vi "JSONtext and SQlite (requires SQLite LabVIEW).vi"() -> ()   [LabVIEW 2017]
uses:
  <vilib>/drjdpowell/SQLite Library/SQL Statement/SQL Statement.lvclass/SQL Statement.ctl
  <vilib>/drjdpowell/SQLite Library/SQL Connection/Open (path).vi
  <vilib>/drjdpowell/SQLite Library/SQL Statement/Bind UTF-8 Text.vi
  a4ef3bbe-680b-444f-9f5b-3aba932734da.vi
  <vilib>/drjdpowell/SQLite Library/SQL Statement/Bind Integer.vi
  <vilib>/drjdpowell/SQLite Library/SQL Connection/Open (string).vi
  <vilib>/AdvancedString/Path To Command Line String.vi
  <vilib>/drjdpowell/SQLite Library/SQL Connection/Execute SQL (No results).vi
  <vilib>/drjdpowell/SQLite Library/SQL Statement/Error Message.vi
  <vilib>/drjdpowell/SQLite Library/SQL Connection/Execute SQL (Single DBL).vi
  <vilib>/drjdpowell/SQLite Library/SQL Statement/Column UTF-8 Text.vi
  JSON text to Variant.vi
  <vilib>/drjdpowell/SQLite Library/SQL Connection/Connection.lvclass
  JSONtext.lvlib
  <vilib>/drjdpowell/SQLite Library/SQLite.lvlib
  <vilib>/drjdpowell/SQLite Library/SQL Statement/SQL Statement.lvclass
  <vilib>/drjdpowell/SQLite Library/Transaction Helpers/Transaction.lvlib
panel:
  out "Average Age":dbl format="%#.6g"
  out "Returned":cluster{string, dbl, string}[](array[cluster]) caption="Returned people of that age" {"?" format="%#_f"}
  in  "Age":i64=32
  # "This example requires both JSONtext and \"SQLite LabVIEW\" packages"
  # "http://sine.ni.com/nips/cds/view/p/lang/en/nid/212894"
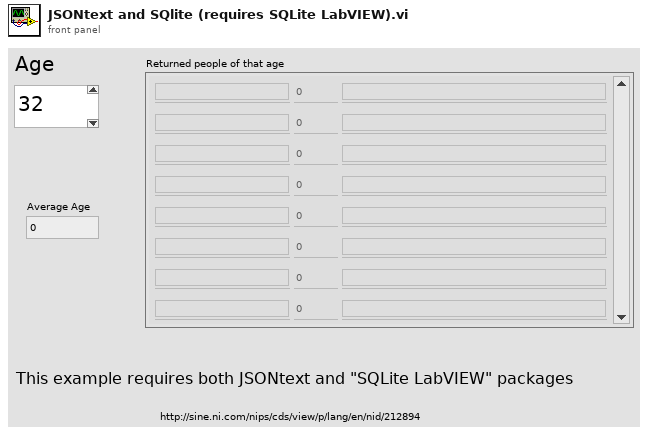
[diagram p1: front panel]
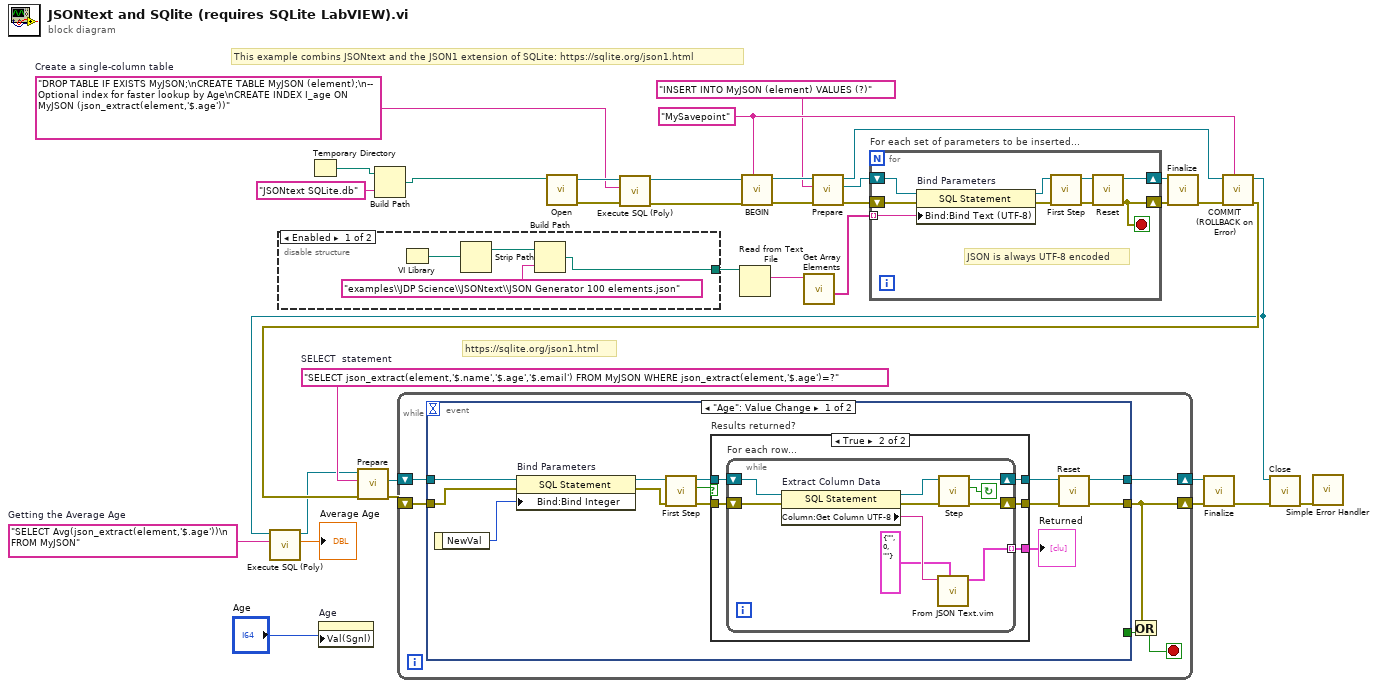
[diagram p0: block diagram]
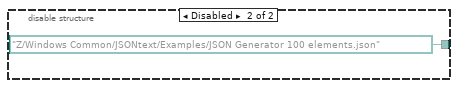
[diagram p2: hidden frame]
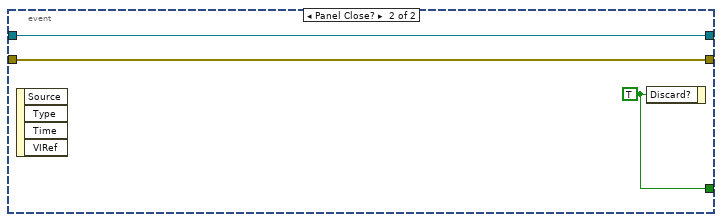
[diagram p4: hidden frame]
diagram:
  w6 = "SELECT Avg(json_extract(element,'$.age'))\n FROM MyJSON"  # Getting the Average Age
  w14 = "SELECT json_extract(element,'$.name','$.age','$.email') FROM MyJSON WHERE json_extract(element,'$.age')=?"  # SELECT  statement
  w29 = "MySavepoint" ("Savepoint name")
  w32 = "DROP TABLE IF EXISTS MyJSON;\nCREATE TABLE MyJSON (element);\n-- Optional index for faster lookup by Age\nCREATE INDEX I_age ON MyJSON (json_extract(element,'$.age'))"  # Create a single-column table
  # "This example combins JSONtext and the JSON1 extension of SQLite: https://sqlite.org/json1.html"
  # "https://sqlite.org/json1.html"
  n1 = disable-structure shown="Enabled" {
    disable-tunnel: [w35 path "Z:/Windows Common/JSONtext/Examples/JSON Generator 100 elements.json" ("appended path")] -> w1
    frame Enabled {
      n2 = VI Library() -> (path=w37:path)
      n3 = Strip Path(path=w37) -> (stripped path=w38:path)  [unwired: 1 out]
      n4 = Build Path(base path=w38, name or relative path="examples\\JDP Science\\JSONtext\\JSON Generator 100 elements.json") -> (appended path=w35:path)
    }
    frame Disabled {
    }
  }
  n5 = Temporary Directory() -> (w4:path)
  n6 = property on="Age" class="DigNum (strict)"("Val(Sgnl)"="Age") -> ()  [unwired: 2 in, 2 out]
  n7 = Build Path(base path=w4, name or relative path="JSONtext SQLite.db") -> (appended path=w2:path)
  n8 = call-poly <vilib>:"Open.vi"("db file"=w2) -> ("error out"=w19:errorcluster, "SQLite Connection"=w33:refnum<class "Connection.lvclass">)  [unwired: 9 in]
  n9 = call-poly <vilib>:"Execute SQL (Poly).vi"("error in (no error)"=w19, "SQL"=w32, "SQLite Connection in"=w33) -> ("error out"=w18:errorcluster, "SQLite Connection"=w20:refnum<class "Connection.lvclass">)  [unwired: 7 in]
  n10 = Read from Text File(file (use dialog)=w1) -> (text=w34:string)  [unwired: 3 in, 3 out]
  n11 = call <vilib>:"BEGIN.vi"("Savepoint name"=w29, "error in (no error)"=w18, "SQLite Connection in"=w20) -> ("error out"=w28:errorcluster, "SQLite Connection"=w27:refnum<class "Connection.lvclass">)  [unwired: 7 in]
  n12 = call "Get Array Elements.vi"("JSON"=w34) -> ("<JSON>"=w21:string[])  [unwired: 8 in, 2 out]
  n13 = call <vilib>:"Prepare.vi"("error in (no error)"=w28, "SQL"="INSERT INTO MyJSON (element) VALUES (?)" ("INSERT statement"), "SQLite Connection in"=w27) -> ("error out"=w23:errorcluster, "SQL Statement"=w22:refnum<class "SQL Statement.lvclass">, "SQLite Connection"=w30:refnum<class "Connection.lvclass">)  [unwired: 4 in, 2 out]
  n14 = for "For each set of parameters to be inserted..." {
    shift-right: [w42] -> w25
    shift-left: w22 -> [w48]
    shift-right: [w41] -> w26
    shift-left: w23 -> [w45]
    tunnel: w21 -> [w40] mode=indexing
    stop <- w41 stop-if-true
    # "JSON is always UTF-8 encoded"
    n15 = property on="Bind Parameters" class="SQL Statement"(reference=w48, error in=w45, "Bind:Bind Text (UTF-8)"=w40) -> (reference out=w47:refnum<class "SQL Statement.lvclass">, error out=w46:errorcluster)
    n16 = call <vilib>:"First Step.vi"("error in (no error)"=w46, "SQL Statement in"=w47) -> ("error out"=w44:errorcluster, "SQL Statement"=w43:refnum<class "SQL Statement.lvclass">)  [unwired: 7 in, 1 out]
    n17 = call <vilib>:"Reset.vi"("error in (no error)"=w44, "SQL Statement in"=w43) -> ("error out"=w41:errorcluster, "SQL Statement"=w42:refnum<class "SQL Statement.lvclass">)  [unwired: 8 in]
  }
  n18 = call <vilib>:"Finalize.vi"("error in (no error)"=w26, "SQL Statement in"=w25) -> ("error out"=w31:errorcluster)  [unwired: 9 in]
  n19 = call <vilib>:"COMMIT (ROLLBACK on Error).vi"("Savepoint name"=w29, "error in (no error)"=w31, "SQLite Connection in"=w30) -> ("error out"=w10:errorcluster, "SQLite Connection"=w7:refnum<class "Connection.lvclass">)  [unwired: 7 in]
  n20 = call-poly <vilib>:"Execute SQL (Poly).vi"("SQL"=w6, "SQLite Connection in"=w7) -> ("Result"=→"Average Age":dbl, "SQLite Connection"=w8:refnum<class "Connection.lvclass">)  [unwired: 7 in, 1 out]
  n21 = call <vilib>:"Prepare.vi"("error in (no error)"=w10, "SQL"=w14, "SQLite Connection in"=w8) -> ("error out"=w13:errorcluster, "SQL Statement"=w12:refnum<class "SQL Statement.lvclass">)  [unwired: 4 in, 3 out]
  n22 = while {
    shift-right: [w49] -> w16
    shift-left: w13 -> [w53]
    shift-right: [w54] -> w15
    shift-left: w12 -> [w52]
    stop <- w50 stop-if-true
    n23 = event shown="[0] \"Age\": Value Change" {
      selector: _ -> [_ _]
      dyn-events: _ -> [_ _]
      timeout: _ -> [_ _]
      tunnel: [w57 w85] -> w49
      tunnel: [w56 w86] -> w54
      tunnel: w53 -> [w67 w85]
      tunnel: w52 -> [w64 w86]
      tunnel: [_ w87] -> w51
      event "Age": Value Change {
        n24 = event-data() -> ("NewVal"=w60:i64)  [unwired: 1 in]
        n25 = property on="Bind Parameters" class="SQL Statement"(reference=w64, error in=w67, "Bind:Bind Integer"=w60) -> (reference out=w65:refnum<class "SQL Statement.lvclass">, error out=w66:errorcluster)
        n26 = call <vilib>:"First Step.vi"("error in (no error)"=w66, "SQL Statement in"=w65) -> ("error out"=w62:errorcluster, "Row returned"=w61:bool, "SQL Statement"=w63:refnum<class "SQL Statement.lvclass">)  [unwired: 7 in]
        n27 = case "Results returned?" shown="True" w61 {
          tunnel: [w69 w74] -> w58
          tunnel: [w68 w73] -> w59
          tunnel: w63 -> [w69 w72]
          tunnel: w62 -> [w68 w71]
          tunnel: [_ w70] -> w55
          frame False {
          }
          frame True {
            n28 = while "For each row..." {
              shift-right: [w83] -> w74
              shift-left: w72 -> [w80]
              shift-right: [w81] -> w73
              shift-left: w71 -> [w79]
              tunnel: [w75] -> w70 mode=indexing
              stop <- w78 continue-if-true
              n29 = property on="Extract Column Data" class="SQL Statement"(reference=w80, error in=w79) -> (reference out=w84:refnum<class "SQL Statement.lvclass">, error out=w82:errorcluster, "Column:Get Column UTF-8"=w77:string)
              n30 = call "From JSON Text.vim"("Data Type and Default Value"=cluster{string, i32, string} {"", 0, ""}, "JSON"=w77) -> ("Data out"=w75:cluster{string, i32, string})  [unwired: 8 in, 1 out]
              n31 = call <vilib>:"Step.vi"("error in (no error)"=w82, "SQL Statement in"=w84) -> ("error out"=w81:errorcluster, "Row returned"=w78:bool, "SQL Statement"=w83:refnum<class "SQL Statement.lvclass">)  [unwired: 7 in]
            }
          }
        }
        "Returned" <- w55
        n32 = call <vilib>:"Reset.vi"("error in (no error)"=w59, "SQL Statement in"=w58) -> ("error out"=w57:errorcluster, "SQL Statement"=w56:refnum<class "SQL Statement.lvclass">)  [unwired: 8 in]
      }
      event Panel Close? {
        w87 = TRUE ("Discard?")
        n33 = event-data() -> ()  [unwired: 1 in, 4 out]
        n34 = event-data("Discard?"=w87) -> ()  [unwired: 1 in, 1 out]
      }
    }
    n35 = Or(x=w49, y=w51) -> (x .or. y?=w50:bool)
  }
  n36 = call <vilib>:"Finalize.vi"("error in (no error)"=w16, "SQL Statement in"=w15) -> ("error out"=w11:errorcluster)  [unwired: 9 in]
  n37 = call-dynamic "Close.vi"("error in (no error)"=w11, "SQLite Connection in"=w7) -> ("error out"=w17:errorcluster)  [unwired: 9 in]
  n38 = call <vilib>:"Simple Error Handler.vi"("error in (no error)"=w17) -> ()  [unwired: 4 in, 5 out]
